vi "Reset User Interface.vi"(8 "error in (no error)":errorcluster, 11 "Sequencer in":refnum<class "Sequencer.lvclass">) -> (0 "error out":errorcluster, 3 "Sequencer out":refnum<class "Sequencer.lvclass">)   [LabVIEW 2024, in "Ramses Sequencer.lvlib" / "Sequencer.lvclass"]
uses:
  Sequencer.lvclass
  Base Step/Base Step.lvclass/Base Step.ctl
  Base Step/Public API/Set Property.vi
  Sequence/Sequence.lvclass
  Base Step/Base Step.lvclass
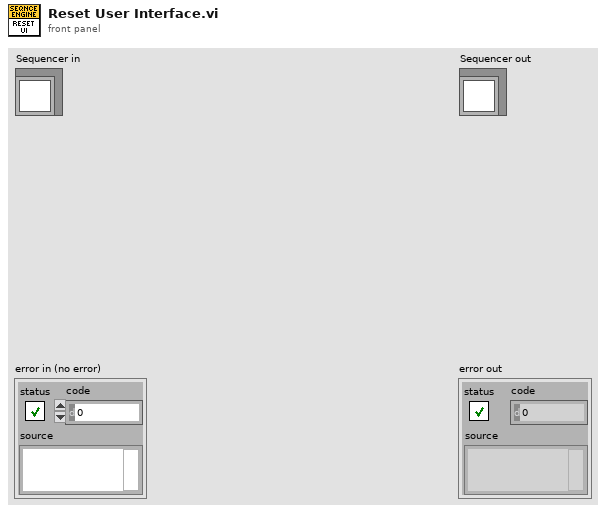
[diagram p1: front panel]
types:
  T1 = typedef "Ramses Sequencer.lvlib/Base Step.lvclass/Step State.ctl" = cluster{"Result":string, "Status":string, "Enabled":bool, "Upper":string, "Target":string, "Lower":string, "Value":string}
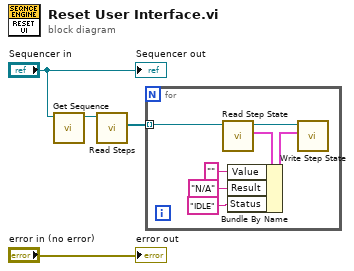
[diagram p0: block diagram]
diagram:
  n1 = call "Get Sequence.vi"("Sequencer in"="Sequencer in") -> ("Sequence"=w4:refnum<class "Sequence.lvclass">)  [unwired: 9 in, 1 out]
  n2 = call-dynamic "Read Steps.vi"("Sequence in"=w4) -> ("Steps"=w3:refnum<class "Base Step.lvclass">[])  [unwired: 8 in, 2 out]
  n3 = for {
    tunnel: w3 -> [w8] mode=indexing
    n4 = call "Read Step State.vi"("Base Step in"=w8) -> ("Step State"=w7:T1, "Base Step out"=w6:refnum<class "Base Step.lvclass">)  [unwired: 8 in, 1 out]
    n5 = Bundle By Name(cluster=w7, "Value"="", "Result"="N/A", "Status"="IDLE" ("Result")) -> (w5:T1)
    n6 = call "Write Step State.vi"("Step State"=w5, "Base Step in"=w6) -> ()  [unwired: 8 in, 2 out]
  }
  "error out" <- "error in (no error)"
  "Sequencer out" <- "Sequencer in"
